vi "манчестер декодер (SubVI).vi"(11 "Кодированные данные":bool[](array[boolean])) -> (3 "Декодированные данные":bool[](array[boolean]))   [LabVIEW 2015]
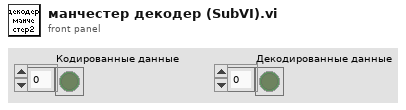
[diagram p1: front panel]
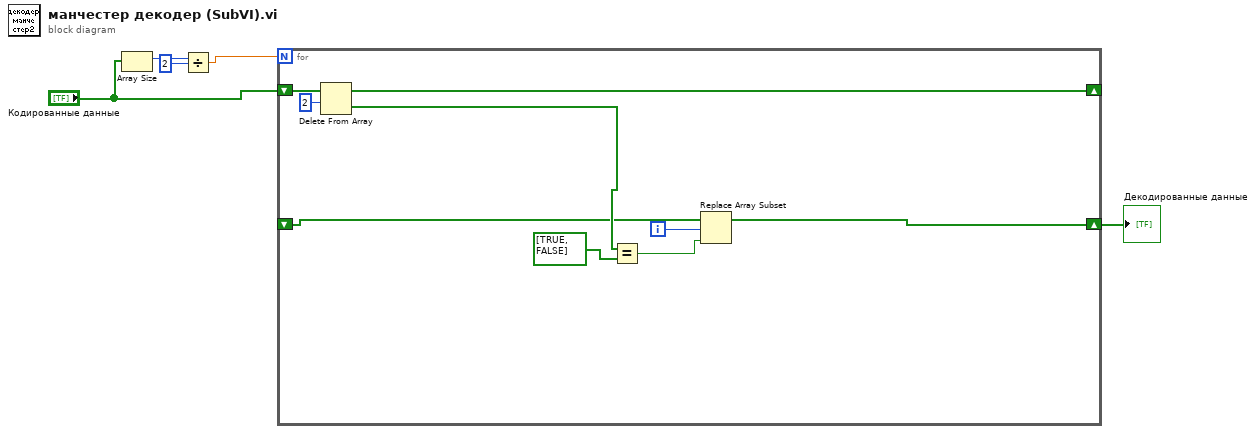
[diagram p0: block diagram]
diagram:
  n1 = Array Size(array="Кодированные данные") -> (size(s)=w3:i32)
  n2 = Divide(x=w3, y=2) -> (x/y=w1:dbl)
  n3 = for {
    N: w1 -> [_]
    shift-right: [w12] -> _
    shift-left: "Кодированные данные" -> [w14]
    shift-right: [w13] -> w5
    shift-left: _ -> [w7]
    i -> [w6]
    n4 = Delete From Array(array=w14, length=2) -> (deleted portion=w9:bool[], array with subset deleted=w12:bool[])  [unwired: 1 in]
    n5 = Equal?(x=w9, y=bool[] [TRUE, FALSE]) -> (x = y?=w8:bool)
    n6 = Replace Array Subset(array=w7, new element=w8, index=w6) -> (w13:bool[])
  }
  "Декодированные данные" <- w5
